vi "Tab_002_PH.vi"() -> ()   [LabVIEW 2021]
panel:
  out "Utworzona tablica":dbl[](array[numeric])=[3.4000000000000004, 3.4000000000000004, 3.4000000000000004, 3.4000000000000004, 3.4000000000000004, 3.4000000000000004]
  in  "Wartoœæ elementów tablicy":dbl=3.4000000000000004
  in  "Liczba elementów tablicy":i32=6
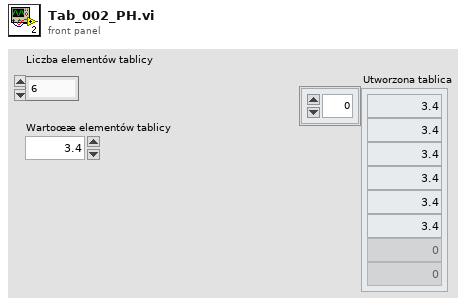
[diagram p1: front panel]
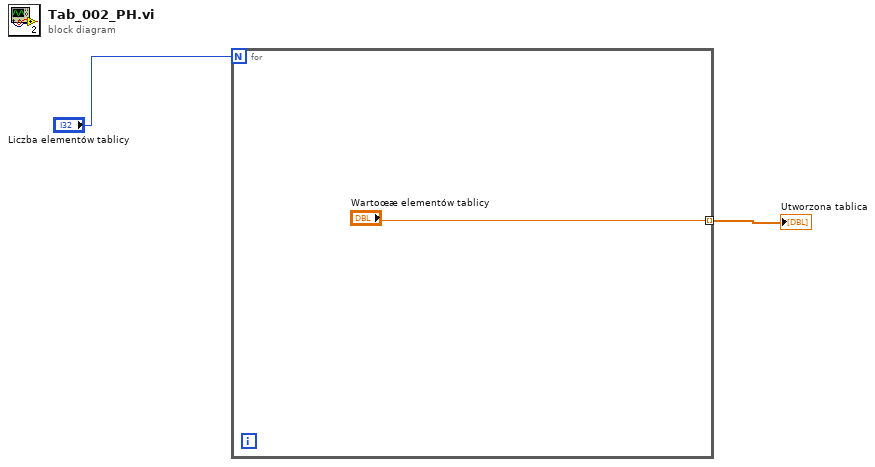
[diagram p0: block diagram]
diagram:
  n1 = for {
    N: "Liczba elementów tablicy" -> [_]
    tunnel: ["Wartoœæ elementów tablicy"] -> w1 mode=indexing
  }
  "Utworzona tablica" <- w1
